vi "conventional fft rep.vi"(2 "Deg/Rad":enum16{"Rad", "Deg"}(ring), 3 "samples":i32=128, 4 "Phase correction":bool, 5 "Phase Unwrap":bool, 6 "fundamental frequency":dbl, 7 "fft output":cdb[](array[numeric])) -> (0 "Conventional FFT phase":cluster{dbl, "fundamental frequency":dbl, dbl[]}, 1 "Conventional FFT mag":cluster{dbl, "fundamental frequency":dbl, dbl[]})   [LabVIEW 2009]
uses:
  <vilib>/Analysis/NI_AALPro.lvlib
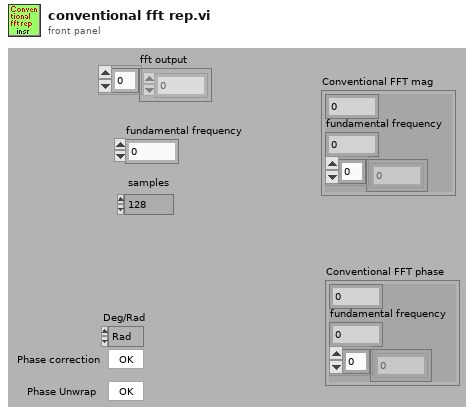
[diagram p1: front panel]
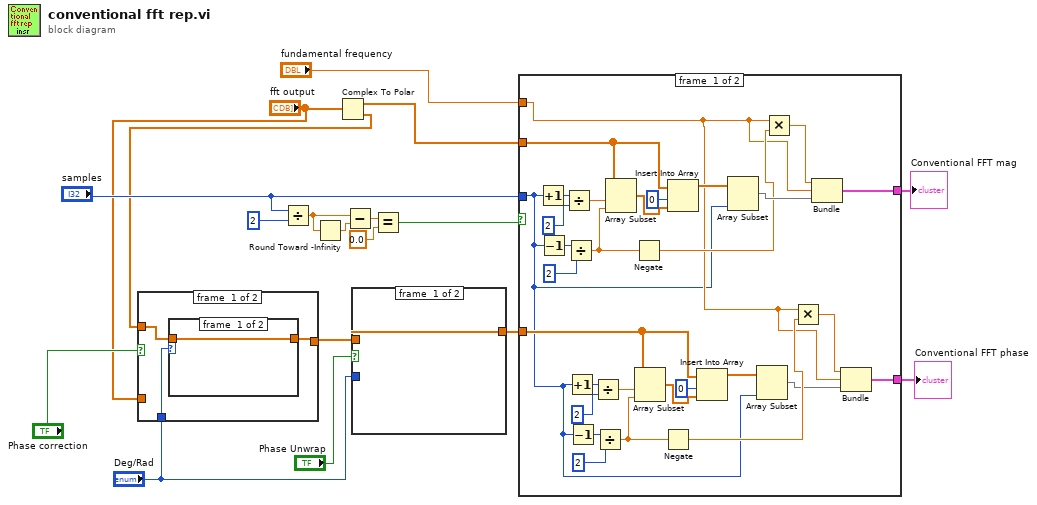
[diagram p0: block diagram]
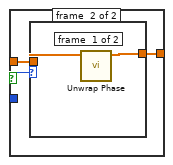
[diagram p2: hidden frame]
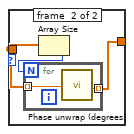
[diagram p3: hidden frame]
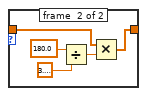
[diagram p4: hidden frame]
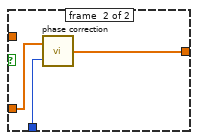
[diagram p5: hidden frame]
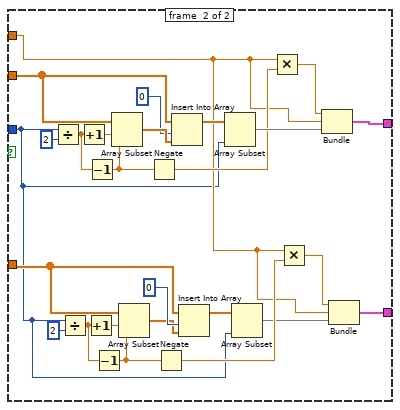
[diagram p6: hidden frame]
diagram:
  n1 = Divide(x="samples", y=2) -> (x/y=w16:dbl)
  n2 = Round Toward -Infinity(1:w16) -> (0:w17:dbl)
  n3 = Complex To Polar(r * e^(i*theta)="fft output") -> (r=w12:dbl[], theta=w4:dbl[])
  n4 = case shown="False" "Phase correction" {
    tunnel: [w19 w30] -> w5
    tunnel: w4 -> [w20 _]
    tunnel: "fft output" -> [_ w29]
    tunnel: "Deg/Rad" -> [w21 w28]
    frame #0 {
      n5 = case shown="\"Rad\", Default" w21 {
        tunnel: w20 -> [w22 w24]
        tunnel: [w22 w23] -> w19
        frame #0 {
        }
        frame #1 {
          n6 = Divide(x=180.0 ("y"), y=3.141592653589793) -> (x/y=w27:dbl)
          n7 = Multiply(x=w24, y=w27) -> (x*y=w23:dbl[])
        }
      }
    }
    frame #1 {
      n8 = call "phase correction.vi"("Deg/Rad"=w28, "Complex FFT"=w29) -> ("Phase"=w30:dbl[])
    }
  }
  n9 = Subtract(x=w16, y=w17) -> (x-y=w15:dbl)
  n10 = case shown="True" "Phase Unwrap" {
    tunnel: [w31 w34] -> w7
    tunnel: w5 -> [w31 w33]
    tunnel: "Deg/Rad" -> [_ w32]
    frame #0 {
    }
    frame #1 {
      n11 = case shown="\"Deg\"" w32 {
        tunnel: [w36 w37] -> w34
        tunnel: w33 -> [w35 w38]
        frame #0 {
          n12 = call <vilib>:"Unwrap Phase.vi"("Phase"=w35) -> ("Unwrapped Phase"=w36:dbl[])  [unwired: 9 in, 1 out]
        }
        frame #1 {
          n13 = Array Size(array=w38) -> (size(s)=w39:i32)
          n14 = for {
            N: w39 -> [_]
            tunnel: w38 -> [w41] mode=indexing
            tunnel: [w40] -> w37 mode=indexing
            n15 = call "Phase unwrap (degrees).vi"("Phase Shift (phy)\n(degrees)"=w41) -> ("Degree"=w40:dbl)
          }
        }
      }
    }
  }
  n16 = Equal?(x=w15, y=0.0) -> (x = y?=w13:bool)
  n17 = case shown="True" w13 {
    tunnel: w12 -> [w66 w94]
    tunnel: "samples" -> [w43 w73]
    tunnel: [w60 w88] -> w9
    tunnel: "fundamental frequency" -> [w44 w74]
    tunnel: w7 -> [w45 w75]
    tunnel: [w42 w72] -> w8
    frame #0 {
      n18 = Increment(x=w43) -> (x+1=w71:i32)
      n19 = Decrement(x=w43) -> (x-1=w68:i32)
      n20 = Divide(x=w71, y=2) -> (x/y=w69:dbl)
      n21 = Divide(x=w68, y=2) -> (x/y=w61:dbl)
      n22 = Increment(x=w43) -> (x+1=w46:i32)
      n23 = Decrement(x=w43) -> (x-1=w49:i32)
      n24 = Divide(x=w46, y=2) -> (x/y=w48:dbl)
      n25 = Divide(x=w49, y=2) -> (x/y=w55:dbl)
      n26 = Array Subset(array=w66, index=w69, length=w61) -> (w64:dbl[])
      n27 = Negate(x=w61) -> (-x=w59:dbl)
      n28 = Array Subset(array=w45, index=w48, length=w55) -> (w52:dbl[])
      n29 = Negate(x=w55) -> (-x=w56:dbl)
      n30 = Insert Into Array(array=w66, index=0, new element=w64) -> (w63:dbl[])
      n31 = Insert Into Array(array=w45, index=0, new element=w52) -> (w53:dbl[])
      n32 = Array Subset(array=w63, length=w43) -> (w62:dbl[])  [unwired: 1 in]
      n33 = Array Subset(array=w53, length=w43) -> (w54:dbl[])  [unwired: 1 in]
      n34 = Multiply(x=w44, y=w59) -> (x*y=w58:dbl)
      n35 = Multiply(x=w44, y=w56) -> (x*y=w57:dbl)
      n36 = Bundle(w58, "fundamental frequency"=w44, w62) -> (w60:cluster{dbl, "fundamental frequency":dbl, dbl[]})  [unwired: 1 in]
      n37 = Bundle(w57, "fundamental frequency"=w44, w54) -> (w42:cluster{dbl, "fundamental frequency":dbl, dbl[]})  [unwired: 1 in]
    }
    frame #1 {
      n38 = Divide(x=w73, y=2) -> (x/y=w95:dbl)
      n39 = Divide(x=w73, y=2) -> (x/y=w78:dbl)
      n40 = Increment(x=w95) -> (x+1=w96:dbl)
      n41 = Increment(x=w78) -> (x+1=w77:dbl)
      n42 = Decrement(x=w95) -> (x-1=w89:dbl)
      n43 = Decrement(x=w78) -> (x-1=w83:dbl)
      n44 = Array Subset(array=w94, index=w96, length=w89) -> (w93:dbl[])
      n45 = Array Subset(array=w75, index=w77, length=w83) -> (w79:dbl[])
      n46 = Negate(x=w89) -> (-x=w87:dbl)
      n47 = Negate(x=w83) -> (-x=w84:dbl)
      n48 = Insert Into Array(array=w94, index=0, new element=w93) -> (w91:dbl[])
      n49 = Insert Into Array(array=w75, index=0, new element=w79) -> (w81:dbl[])
      n50 = Array Subset(array=w91, length=w73) -> (w90:dbl[])  [unwired: 1 in]
      n51 = Array Subset(array=w81, length=w73) -> (w82:dbl[])  [unwired: 1 in]
      n52 = Multiply(x=w74, y=w87) -> (x*y=w86:dbl)
      n53 = Multiply(x=w74, y=w84) -> (x*y=w85:dbl)
      n54 = Bundle(w86, "fundamental frequency"=w74, w90) -> (w88:cluster{dbl, "fundamental frequency":dbl, dbl[]})  [unwired: 1 in]
      n55 = Bundle(w85, "fundamental frequency"=w74, w82) -> (w72:cluster{dbl, "fundamental frequency":dbl, dbl[]})  [unwired: 1 in]
    }
  }
  "Conventional FFT mag" <- w9
  "Conventional FFT phase" <- w8
